vi "generalized projections.vi"() -> ()   [LabVIEW 2013]
uses:
  <vilib>/Analysis/2dsp.llb/Complex FFT.vi
  <vilib>/Analysis/2dsp.llb/Inverse Complex FFT.vi
  <vilib>/Analysis/NI_AALPro.lvlib
panel:
  out "Present Err":dbl format="%#_3g"
  in  "Target Err":dbl=5e-06
  out "Itr Count":u16
  in  "Max Itr":u16=5000
  out "Spectrum":cluster{ext[], dbl[]}[](graph)
  out "Error Chart":dbl(graph)
  out "Temporal Signal":cluster{"Time Array":dbl[], "Noise Array":dbl[]}(graph)
  out "Recovered Trace":dbl[][](graph)
  in  "Delay Info":T1
  in  "Spectrum Info":T2
  in  "PG Test Data":dbl[][](array[numeric])=array129x256[33024 elements]
  out "Experiment Trace":dbl[][](graph)
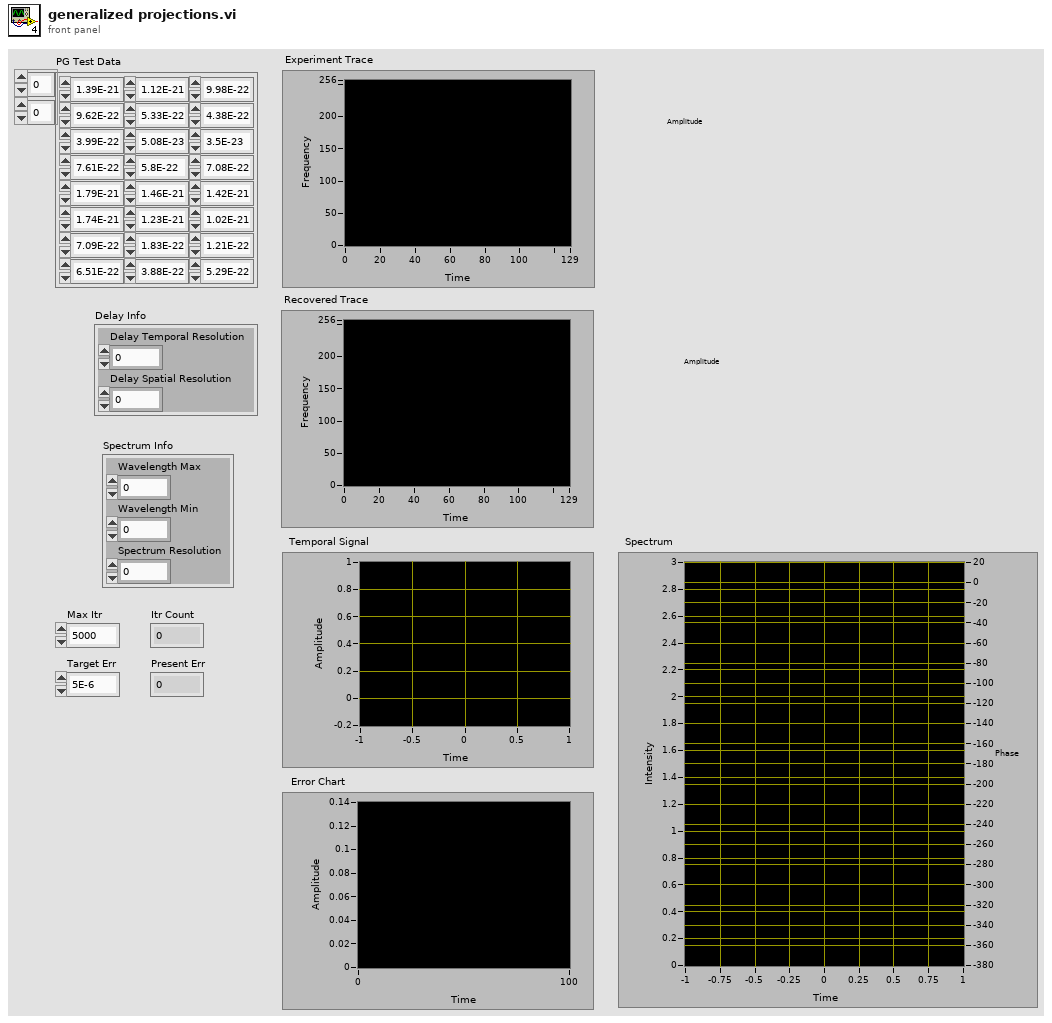
[diagram p1: front panel]
types:
  T1 = cluster{"Delay Temporal Resolution":u16, "Delay Spatial Resolution":u16}
  T2 = cluster{"Wavelength Max":dbl, "Wavelength Min":dbl, "Spectrum Resolution":u16}
  T3 = cluster{"Frequency Max":dbl, "Frequency Min":dbl, "Spectrum Resolution":u16}
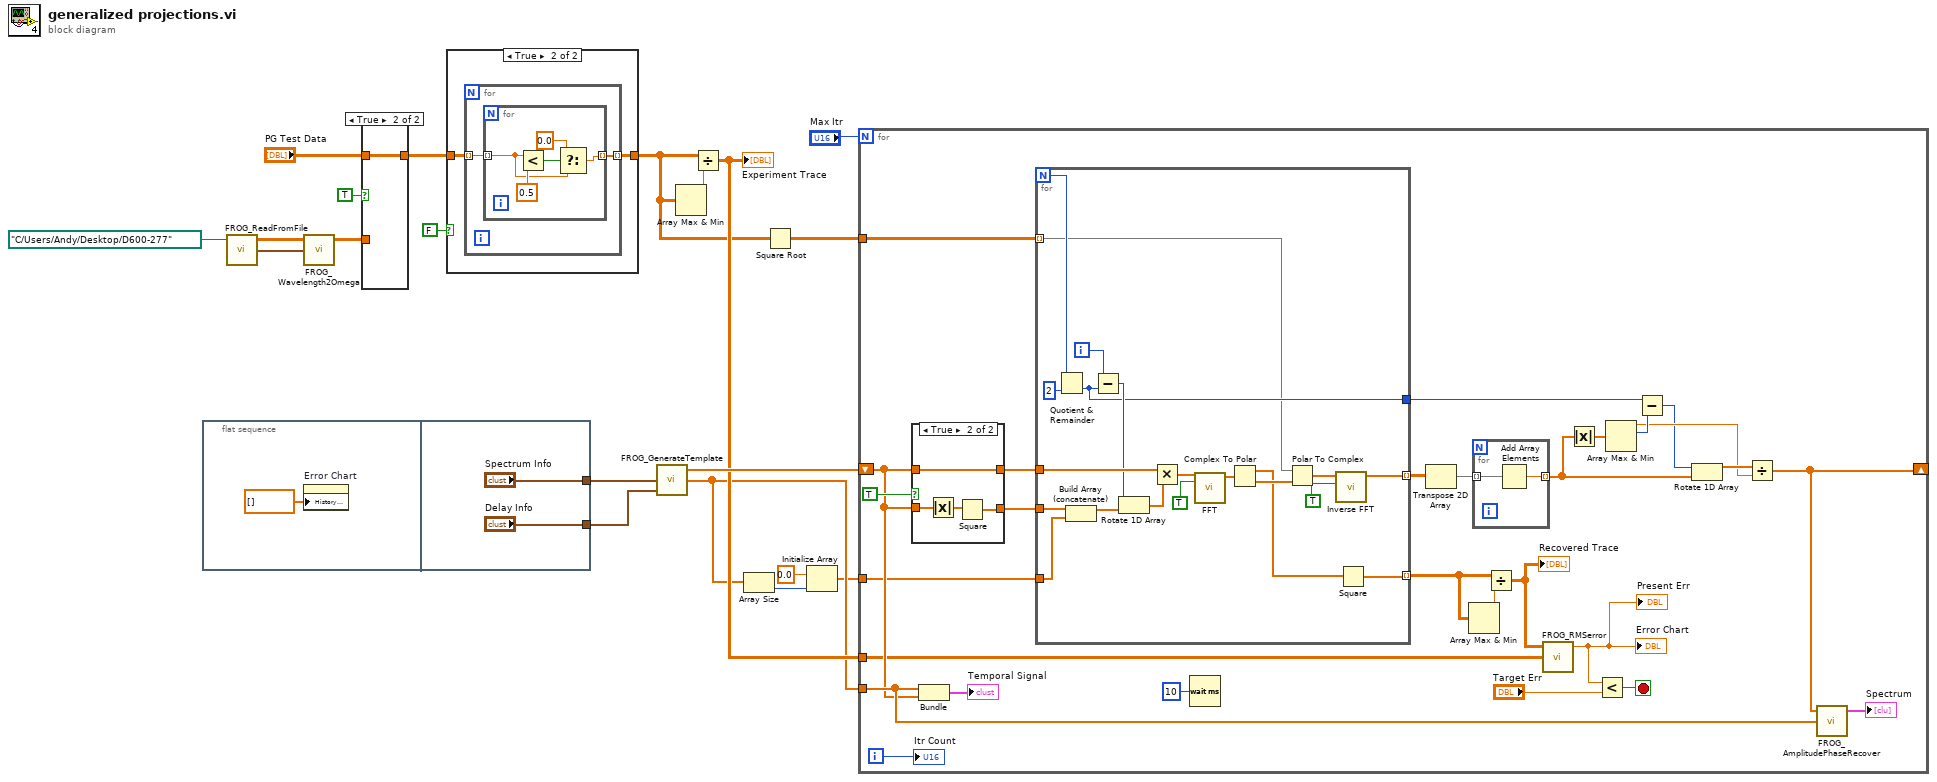
[diagram p0: block diagram]
diagram:
  n1 = flat-sequence {
    tunnel: ["Delay Info"] -> w17
    tunnel: ["Spectrum Info"] -> w16
    frame #0 {
      n2 = property on="Error Chart" class="WFChart (strict)"("History Data"=dbl[] []) -> ()  [unwired: 2 in, 2 out]
    }
    frame #1 {
    }
  }
  n3 = call "FROG_ReadFromFile.vi"("File Path"=path "C:/Users/Andy/Desktop/D600-277") -> ("Spectrum Info"=w15:T3, "Experiment Trace"=w19:dbl[][])  [unwired: 2 in, 1 out]
  n4 = call "FROG_Wavelength2Omega.vi"("Spectrum Info"=w15, "Experiment Trace"=w19) -> ("Converted Trace"=w12:dbl[][])  [unwired: 2 in, 1 out]
  n5 = case shown="True" TRUE {
    tunnel: "PG Test Data" -> [_ w25]
    tunnel: [w24 w25] -> w2
    tunnel: w12 -> [w24 _]
    frame False {
    }
    frame True {
    }
  }
  n6 = case shown="True" FALSE {
    tunnel: w2 -> [w26 w28]
    tunnel: [w26 w27] -> w1
    frame False {
    }
    frame True {
      n7 = for {
        tunnel: w28 -> [w30] mode=indexing
        tunnel: [w29] -> w27 mode=indexing
        n8 = for {
          tunnel: w30 -> [w32] mode=indexing
          tunnel: [w31] -> w29 mode=indexing
          n9 = Less?(x=w32, y=0.5) -> (x < y?=w34:bool)
          n10 = Select(t=0.0, s=w34, f=w32) -> (s? t:f=w31:dbl)
        }
      }
    }
  }
  n11 = call "FROG_GenerateTemplate.vi"("Delay Info"=w17, "Spectrum Info"=w16) -> ("Time Array"=w6:dbl[], "Noise Array"=w18:dbl[])  [unwired: 1 in, 1 out]
  n12 = Array Max & Min(array=w1) -> (max value=w14:dbl)  [unwired: 3 out]
  n13 = Divide(x=w1, y=w14) -> (x/y=w9:dbl[][])
  "Experiment Trace" <- w9
  n14 = Array Size(array=w6) -> (size(s)=w5:i32)
  n15 = Square Root(x=w1) -> (sqrt(x)=w10:dbl[][])
  n16 = Initialize Array(0.0 ("element"), w5) -> (w4:dbl[])
  n17 = for {
    N: "Max Itr" -> [_]
    shift-right: [w49] -> _
    shift-left: w18 -> [w51]
    tunnel: w6 -> [w55]
    tunnel: w10 -> [w45]
    tunnel: w9 -> [w44]
    tunnel: w4 -> [w36]
    i -> [w39]
    stop <- w40 stop-if-true
    n18 = case shown="True" TRUE {
      tunnel: [w64 w68] -> w63
      tunnel: w51 -> [w64 w67]
      tunnel: [w65 w66] -> w52
      tunnel: w51 -> [w65 w66]
      frame False {
      }
      frame True {
        n19 = Absolute Value(x=w67) -> (abs(x)=w69:dbl[])
        n20 = Square(x=w69) -> (x^2=w68:dbl[])
      }
    }
    n21 = Bundle("Time Array"=w55, "Noise Array"=w51) -> (→"Temporal Signal":cluster{"Time Array":dbl[], "Noise Array":cdb[]})  [unwired: 1 in]
    n22 = for {
      N -> [w90]
      tunnel: w45 -> [w75] mode=indexing
      tunnel: w52 -> [w89]
      tunnel: w63 -> [w74]
      tunnel: [w81] -> w62 mode=indexing
      tunnel: [w77] -> w46 mode=indexing
      tunnel: [w78] -> w57
      tunnel: w36 -> [w73]
      i -> [w79]
      n23 = Quotient & Remainder(x=w90, y=2) -> (floor(x/y)=w78:i32)  [unwired: 1 out]
      n24 = Build Array (concatenate)(w74, w73) -> (w72:cdb[])
      n25 = Subtract(x=w79, y=w78) -> (x-y=w80:i32)
      n26 = Rotate 1D Array(1:w72, 2:w80) -> (0:w88:cdb[])
      n27 = Multiply(x=w89, y=w88) -> (x*y=w87:cdb[])
      n28 = call-poly <vilib>:"FFT.vi"("shift?"=TRUE, "X"=w87) -> ("FFT {X}"=w85:cdb[])  [unwired: 8 in, 1 out]
      n29 = Complex To Polar(r * e^(i*theta)=w85) -> (r=w76:dbl[], theta=w84:dbl[])
      n30 = Polar To Complex(1:w84, 2:w75) -> (0:w83:cdb[])
      n31 = call-poly <vilib>:"Inverse FFT.vi"("shift?"=TRUE, "FFT {X}"=w83) -> ("X"=w81:cdb[])  [unwired: 8 in, 1 out]
      n32 = Square(x=w76) -> (x^2=w77:dbl[])
    }
    n33 = Wait (ms)(milliseconds to wait=u32 10) -> ()  [unwired: 1 out]
    n34 = Transpose 2D Array(2D array=w62) -> (transposed array=w61:cdb[][])
    n35 = Array Max & Min(array=w46) -> (max value=w48:dbl)  [unwired: 3 out]
    n36 = for {
      tunnel: w61 -> [w70] mode=indexing
      tunnel: [w71] -> w58 mode=indexing
      n37 = Add Array Elements(numeric array=w70) -> (sum=w71:cdb)
    }
    n38 = Divide(x=w46, y=w48) -> (x/y=w47:dbl[][])
    "Recovered Trace" <- w47
    n39 = call "FROG_RMSerror.vi"("Experiment Trace"=w44, "Fit Trace"=w47) -> ("RMS Error"=w37:dbl)  [unwired: 1 in, 2 out]
    "Error Chart" <- w37
    "Present Err" <- w37
    n40 = Absolute Value(x=w58) -> (abs(x)=w59:dbl[])
    n41 = Less?(x=w37, y="Target Err") -> (x < y?=w40:bool)
    n42 = Array Max & Min(array=w59) -> (max value=w42:dbl, max index (indices)=w56:i32)  [unwired: 2 out]
    n43 = Subtract(x=w57, y=w56) -> (x-y=w41:i32)
    n44 = Rotate 1D Array(1:w58, 2:w41) -> (0:w43:cdb[])
    n45 = Divide(x=w43, y=w42) -> (x/y=w49:cdb[])
    n46 = call "FROG_AmplitudePhaseRecover.vi"("Time Array"=w55, "Signal Array"=w49) -> ("Array"=→"Spectrum":cluster{ext[], dbl[]}[])  [unwired: 3 in]
    "Itr Count" <- w39
  }
